vi "Deploy and wait.vi"(8 "error in (no error)":errorcluster, 10 "UUT Path":path, 11 "WorkspaceManager in":T1) -> (0 "error out":errorcluster, 2 "UUT Path dup":path, 3 "WorkspaceManager out":T1)   [LabVIEW 2011]
uses:
  <vilib>/NI Veristand/Execution/Workspace/WorkspaceAPI.ctl
  NationalInstruments.VeriStand.ClientAPI
  <vilib>/NI Veristand/Execution/Workspace/NI_VS Workspace ExecutionAPI.lvlib
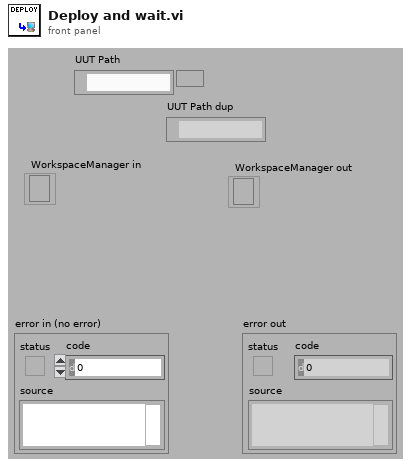
[diagram p1: front panel]
types:
  T1 = typedef "NI_VS Workspace ExecutionAPI.lvlib/WorkspaceAPI.ctl" = refnum<k24>
  T2 = typedef "NI_VS Workspace ExecutionAPI.lvlib/SystemState.ctl" = u8
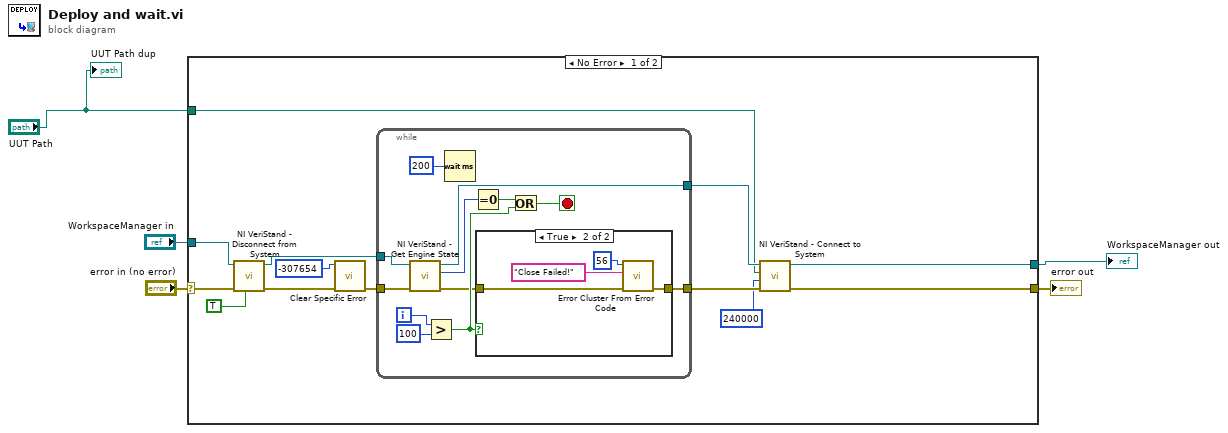
[diagram p0: block diagram]
diagram:
  n1 = case shown="No Error" "error in (no error)" {
    selector: "error in (no error)" -> [w15 w37]
    tunnel: [w10 w37] -> w5
    tunnel: [w11 w36] -> w4
    tunnel: "WorkspaceManager in" -> [w14 w36]
    tunnel: "UUT Path" -> [w16 _]
    frame No Error {
      n2 = call <vilib>:"NI VeriStand - Disconnect from System.vi"("Undeploy System Definition (F)"=TRUE, "error in (no error)"=w15, "WorkspaceManager in"=w14) -> ("error out"=w9:errorcluster, "WorkspaceManager out"=w13:T1)  [unwired: 7 in]
      n3 = call "Clear Specific Error.vi"("error in (no error)"=w9, "code"=-307654) -> ("error out"=w8:errorcluster)  [unwired: 8 in, 1 out]
      n4 = while {
        tunnel: w8 -> [w30]
        tunnel: w13 -> [w29]
        tunnel: [w19] -> w17
        tunnel: [w28] -> w18
        i -> [w25]
        stop <- w22 stop-if-true
        n5 = call <vilib>:"NI VeriStand - Get Engine State.vi"("error in (no error)"=w30, "WorkspaceManager in"=w29) -> ("error out"=w20:errorcluster, "System State"=w26:T2, "WorkspaceManager  out"=w28:T1)  [unwired: 4 in, 3 out]
        n6 = Greater?(x=w25, y=100) -> (0:w21:bool)
        n7 = Wait (ms)(milliseconds to wait=u32 200) -> ()  [unwired: 1 out]
        n8 = Equal To 0?(x=w26) -> (x = 0?=w23:bool)
        n9 = case shown="True" w21 {
          tunnel: [w31 w34] -> w19
          tunnel: w20 -> [w31 w35]
          frame False {
          }
          frame True {
            n10 = call <vilib>:"Error Cluster From Error Code.vi"("error in (no error)"=w35, "error message (\"\")"="Close Failed!" ("error message (\"\")"), "error code (0)"=56) -> ("error out"=w34:errorcluster)  [unwired: 6 in]
          }
        }
        n11 = Or(x=w23, y=w21) -> (x .or. y?=w22:bool)
      }
      n12 = call <vilib>:"NI VeriStand - Connect to System.vi"("error in (no error)"=w17, "Timeout (60000 ms)"=u32 240000, "System Definition File (.nivssdf)"=w16, "WorkspaceManager in"=w18) -> ("error out"=w10:errorcluster, "WorkspaceManager out"=w11:T1)  [unwired: 6 in]
    }
    frame Error {
    }
  }
  "error out" <- w5
  "WorkspaceManager out" <- w4
  "UUT Path dup" <- "UUT Path"
